vi "PDE_Evaluate 2D Func.vi"(7 "data":variant, 8 "error in (no error)":errorcluster, 9 "Y":dbl[](array[numeric]), 10 "X":dbl[](array[numeric]), 11 "VIRef":refnum<vi>) -> (0 "error out":errorcluster, 3 "F(x, y)":dbl[](array[numeric]))   [LabVIEW 2017, in "NI_PDE.lvlib"]
uses:
  <vilib>/gmath/NI_PDE.lvlib
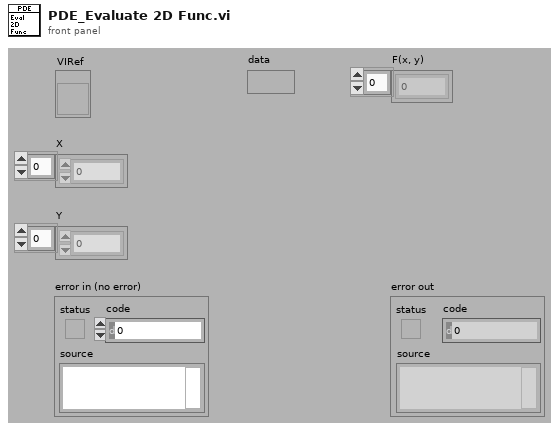
[diagram p1: front panel]
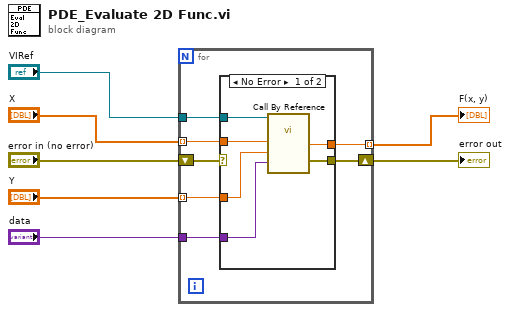
[diagram p0: block diagram]
diagram:
  n1 = for {
    tunnel: "Y" -> [w12] mode=indexing
    tunnel: "VIRef" -> [w14]
    tunnel: "X" -> [w13] mode=indexing
    tunnel: "data" -> [w11]
    shift-right: [w10] -> w5
    shift-left: "error in (no error)" -> [w9]
    tunnel: [w8] -> w3 mode=indexing
    n2 = case shown="No Error" w9 {
      selector: w9 -> [_ w21]
      tunnel: w14 -> [w20 _]
      tunnel: w13 -> [w19 _]
      tunnel: w12 -> [w18 _]
      tunnel: w11 -> [w17 _]
      tunnel: [w16 w21] -> w10
      tunnel: [w15 _] -> w8
      frame No Error {
        n3 = call-by-ref "?"(reference=w20, "data"=w17, "y"=w18, "x"=w19) -> ("error out"=w16:errorcluster, "f(x, y)"=w15:dbl)  [unwired: 1 in, 2 out]
      }
      frame Error {
      }
    }
  }
  "F(x, y)" <- w3
  "error out" <- w5
